vi "Paths to Map.vi"(8 "error in":errorcluster, 10 "Paths":variant, 11 "map in":map{string, map{string, string[]}}(c390)) -> (0 "error out":errorcluster, 3 "map out":map{string, map{string, string[]}}(c390)={"llab_060"={"v000"=["$$X$$"], "v006"=["$$X$$"]}, "llab_061"={"d000"=["0"], "v000"=["$$X$$"], "v003"=["$$X$$"], "v006"=["$$X$$"]}, "llab_063"={"d001"=["5"]}})   [LabVIEW 2019, in "LV-Data.PGSQL.lvclass"]
uses:
  LV-Data.PGSQL.lvclass
  <vilib>/Utility/miscctls.llb/LVMapReplaceAction.ctl
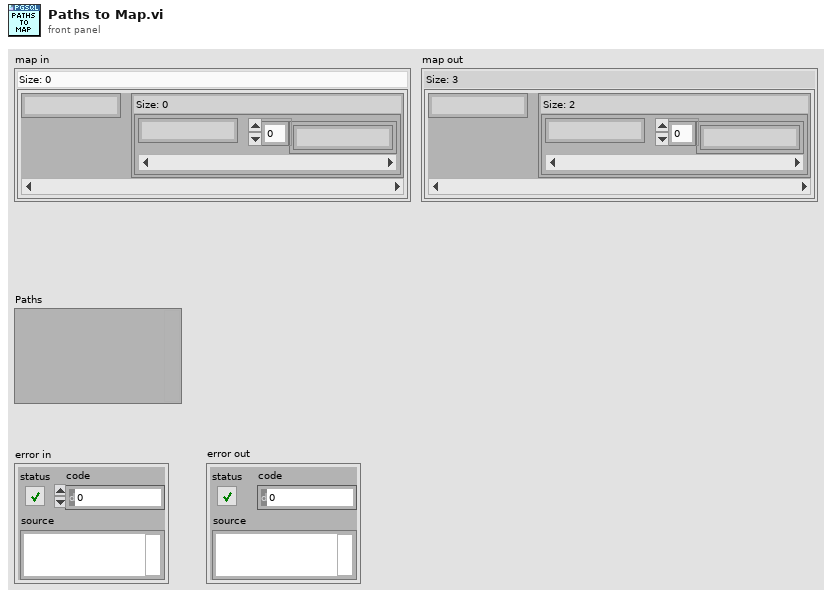
[diagram p1: front panel]
types:
  T1 = typedef "LVMapReplaceAction.ctl" = enum32{"Modify Entry only if found", "Add or Modify Entry", "Delete Entry"}
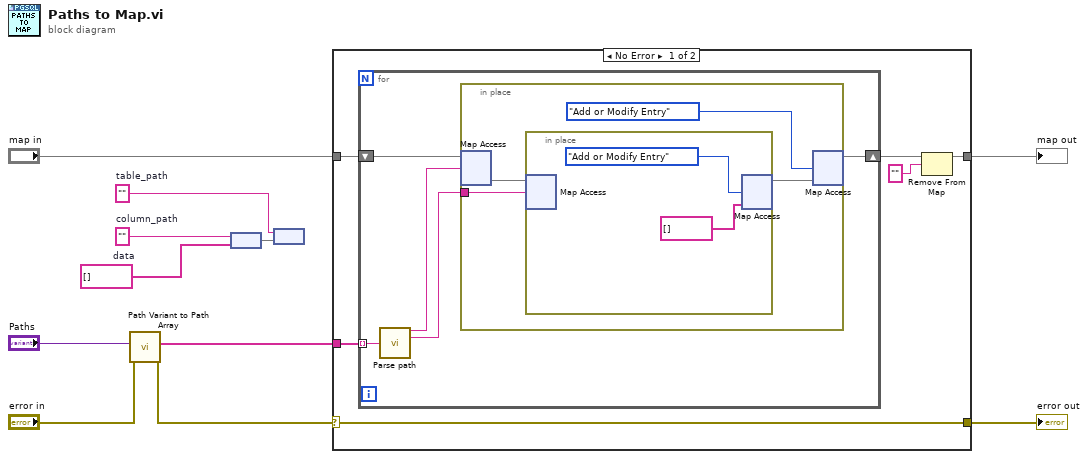
[diagram p0: block diagram]
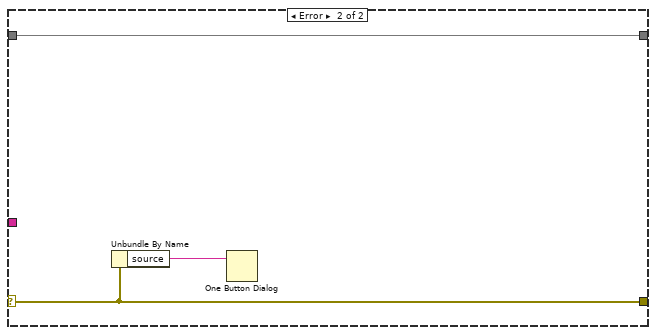
[diagram p2: hidden frame]
diagram:
  w4 = string[] []  # data
  w6 = ""  # column_path
  w5 = ""  # table_path
  n1 = call "Path Variant to Path Array.vi"("error in"="error in", "Paths"="Paths") -> ("error out"=w1:errorcluster, "Paths"=w2:string[])  [unwired: 8 in]
  n2 = node(w6, w4) -> (w7:map{string, string[]})
  n3 = node(w5, w7) -> ()  [unwired: 1 out]
  n4 = case shown="No Error" w1 {
    selector: w1 -> [w12 w30]
    tunnel: "map in" -> [w17 w31]
    tunnel: [w14 w31] -> w11
    tunnel: w2 -> [w13 _]
    tunnel: [w12 w30] -> w10
    frame No Error {
      n5 = for {
        tunnel: w13 -> [w18] mode=indexing
        shift-right: [w19] -> w16
        shift-left: w17 -> [w22]
        n6 = call "Parse path.vi"("PG Path"=w18) -> ("Table path"=w21:string, "Column path"=w20:string)  [unwired: 10 in, 3 out]
        n7 = in-place {
          in-place-border: w20 -> [w25]
          n8 = in-place-map #1(w22, w21) -> (w26:map{string, string[]})  [unwired: 1 in, 1 out]
          n9 = in-place {
            n10 = in-place-map #2(w26, w25) -> ()  [unwired: 1 in, 2 out]
            n11 = in-place-map #2(string[] [], LVMapReplaceAction."Add or Modify Entry" ("action")) -> (w24:map{string, string[]})  [unwired: 2 out]
          }
          n12 = in-place-map #1(w24, LVMapReplaceAction."Add or Modify Entry" ("action")) -> (w19:map{string, map{string, string[]}})  [unwired: 2 out]
        }
      }
      n13 = Remove From Map(10:"" ("key"), 11:w16) -> (3:w14:map{string, map{string, string[]}})  [unwired: 2 out]
    }
    frame Error {
      n14 = Unbundle By Name(w30) -> ("source"=w29:string)
      n15 = One Button Dialog(message=w29) -> ()  [unwired: 1 in, 1 out]
    }
  }
  "error out" <- w10
  "map out" <- w11
